vi "Hypotenuse to Extender Encoder Position.vi"(4 "Extender Enc Pos at 12 inches":dbl, 6 "Min Extender Enc Pos":dbl, 11 "Wanted Extension (Inches)":dbl) -> (2 "Target Extender Enc Pos":dbl)   [LabVIEW 2023]
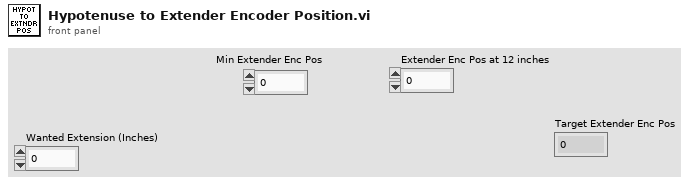
[diagram p1: front panel]
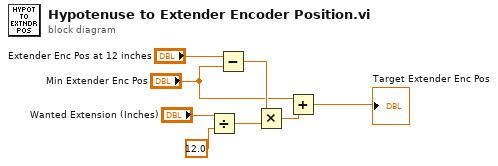
[diagram p0: block diagram]
diagram:
  n1 = Divide(x="Wanted Extension (Inches)", y=12.0) -> (x/y=w5:dbl)
  n2 = Subtract(x="Extender Enc Pos at 12 inches", y="Min Extender Enc Pos") -> (x-y=w4:dbl)
  n3 = Multiply(x=w4, y=w5) -> (x*y=w3:dbl)
  n4 = Add(x="Min Extender Enc Pos", y=w3) -> (x+y=→"Target Extender Enc Pos":dbl)
